vi "App_Auth_handler.vi"(8 "error in (no error)":errorcluster, 10 "Auth Time In":dbl, 11 "Path In":path) -> (0 "error out":errorcluster, 2 "Auth Time Out":dbl, 3 "Cluster":T1, 5 "Path Out":path)   [LabVIEW 2016]
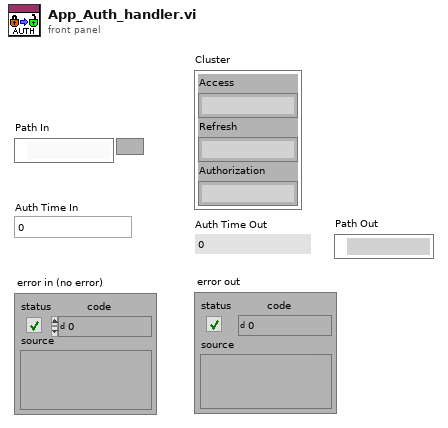
[diagram p1: front panel]
types:
  T1 = cluster{"Access":string, "Refresh":string, "Authorization":string}
  T2 = cluster{"Auth Code Out":string, "Access Token Out":string, "Refresh Token Out":string}
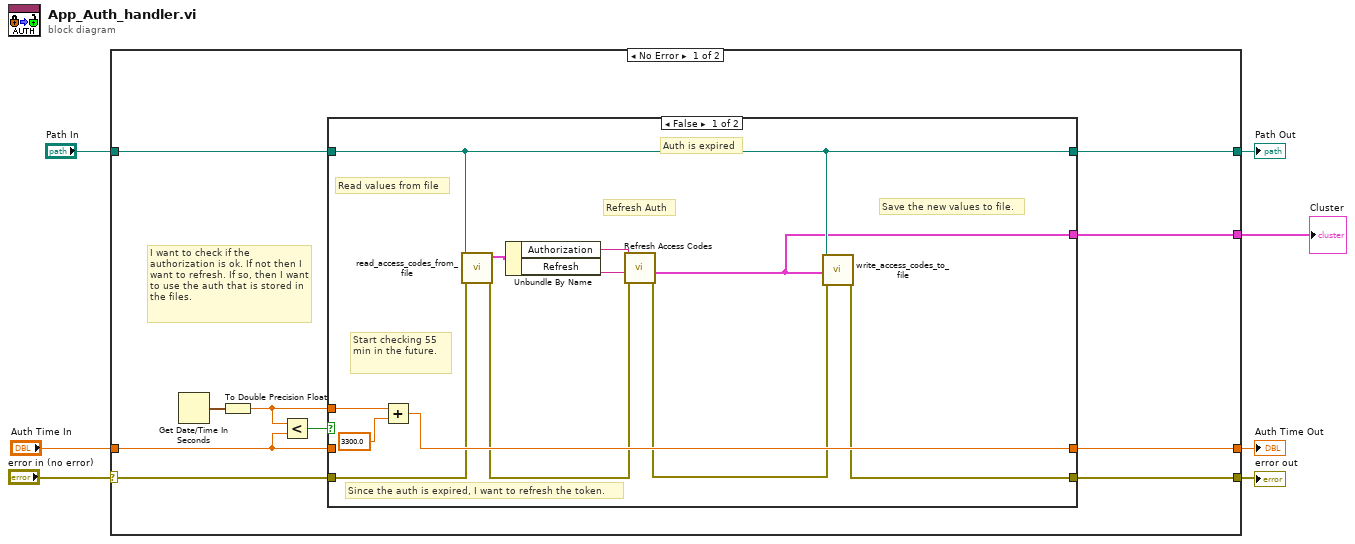
[diagram p0: block diagram]
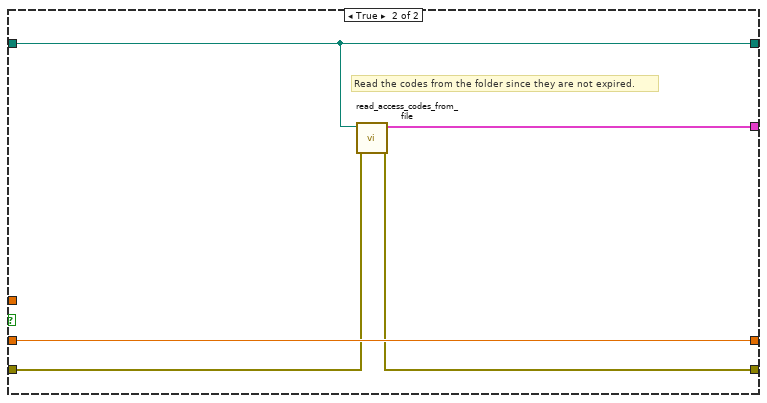
[diagram p2: hidden frame]
diagram:
  n1 = case shown="No Error" "error in (no error)" {
    selector: "error in (no error)" -> [w14 w37]
    tunnel: [w10 w37] -> w6
    tunnel: "Auth Time In" -> [w13 w36]
    tunnel: [w12 w36] -> w4
    tunnel: "Path In" -> [w11 w35]
    tunnel: [w9 w35] -> w2
    tunnel: [w8 _] -> w1
    frame No Error {
      # "I want to check if the authorization is ok. If not then I want to refresh. If so, then I want to use the auth that is stored in the files."
      n2 = Get Date/Time In Seconds() -> (seconds since 1Jan1904=w17:timestamp)
      n3 = To Double Precision Float(number=w17) -> (double precision float=w15:dbl)
      n4 = Less?(x=w15, y=w13) -> (x < y?=w16:bool)
      n5 = case shown="False" w16 {
        tunnel: w13 -> [_ w34]
        tunnel: w15 -> [w29 _]
        tunnel: [w27 w34] -> w12
        tunnel: w14 -> [w25 w32]
        tunnel: w11 -> [w19 w31]
        tunnel: [w20 w33] -> w10
        tunnel: [w19 w31] -> w9
        tunnel: [w18 w30] -> w8
        frame False {
          # "Start checking 55 min in the future."
          # "Refresh Auth"
          # "Read values from file"
          # "Save the new values to file."
          # "Auth is expired"
          # "Since the auth is expired, I want to refresh the token."
          n6 = Add(x=w29, y=3300.0) -> (x+y=w27:dbl)
          n7 = call "read_access_codes_from_file.vi"("error in (no error)"=w25, "Path"=w19) -> ("error out"=w24:errorcluster, "Codes"=w26:T1)  [unwired: 8 in]
          n8 = Unbundle By Name(w26) -> ("Authorization"=w22:string, "Refresh"=w23:string)
          n9 = call "Refresh Access Codes.vi"("error in"=w24, "Refresh Token In"=w23, "Authorization Code In"=w22) -> ("error out"=w21:errorcluster, "Cluster"=w18:T2)  [unwired: 7 in]
          n10 = call "write_access_codes_to_file.vi"("error in (no error)"=w21, "Cluster"=w18, "Path"=w19) -> ("error out"=w20:errorcluster)  [unwired: 8 in]
        }
        frame True {
          # "Read the codes from the folder since they are not expired."
          n11 = call "read_access_codes_from_file.vi"("error in (no error)"=w32, "Path"=w31) -> ("error out"=w33:errorcluster, "Codes"=w30:T1)  [unwired: 8 in]
        }
      }
    }
    frame Error {
    }
  }
  "error out" <- w6
  "Auth Time Out" <- w4
  "Path Out" <- w2
  "Cluster" <- w1
